vi "Read Inner Cost.vi"(11 "Condiment Decorator in":refnum<class "Condiment Decorator.lvclass">) -> (2 "Cost":dbl)   [LabVIEW 2013, in "Condiment Decorator.lvclass"]
uses:
  Condiment Decorator.lvclass
  Condiment Decorator.lvclass/Condiment Decorator.ctl
  Abstract Beverage/Abstract Beverage.lvclass
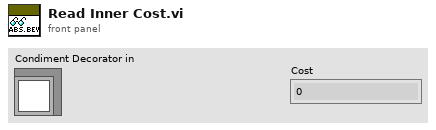
[diagram p1: front panel]
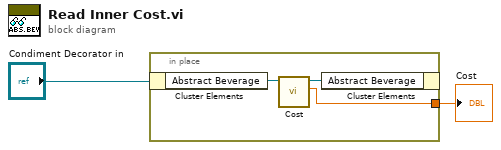
[diagram p0: block diagram]
diagram:
  n1 = in-place {
    in-place-border: [w3] -> w1
    n2 = in-place-cluster #1("Condiment Decorator in") -> ("Abstract Beverage"=w5:refnum<class "Abstract Beverage.lvclass">)
    n3 = call-dynamic "Cost.vi"("Abstract Beverage in"=w5) -> ("Cost"=w3:dbl, "Abstract Beverage out"=w4:refnum<class "Abstract Beverage.lvclass">)  [unwired: 8 in, 1 out]
    n4 = in-place-cluster #1("Abstract Beverage"=w4) -> ()  [unwired: 1 out]
  }
  "Cost" <- w1
